vi "get_speeds_and_positions.vi"(1 "error in (no error)":errorcluster) -> (0 "error out":errorcluster)   [LabVIEW 2016]
uses:
  sa commands.ctl
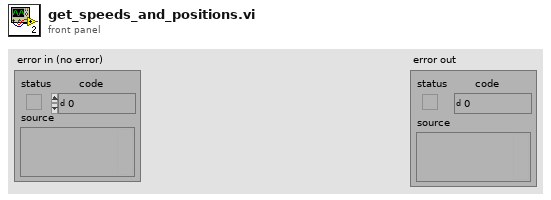
[diagram p1: front panel]
types:
  T1 = typedef "sa commands.ctl" = enum16{"read all", "set system index", "set x channel", "set y channel", "set rotation channel"}
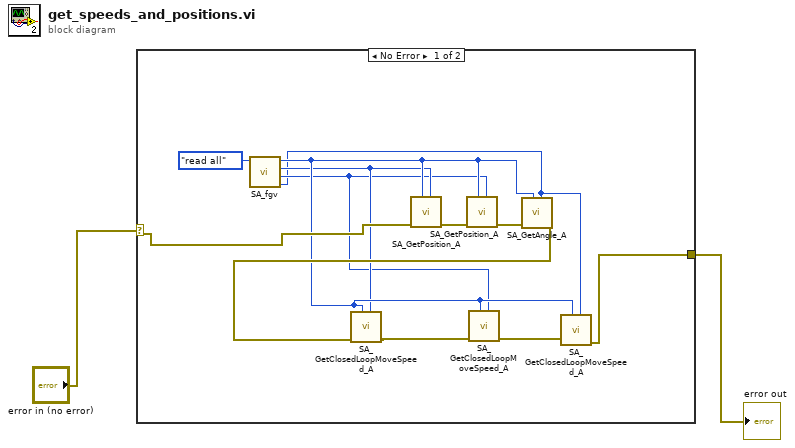
[diagram p0: block diagram]
diagram:
  n1 = case shown="No Error" "error in (no error)" {
    selector: "error in (no error)" -> [w11 w15]
    tunnel: [w3 w15] -> w1
    frame No Error {
      n2 = call "SA_fgv.vi"("command"=sa_commands."read all") -> ("rotation channel"=w4:u32, "y channel"=w5:u32, "x channel"=w6:u32, "system index"=w7:u32)  [unwired: 3 in]
      n3 = call <vilib>:"SA_GetPosition_A.vi"("channelIndex"=w6, "systemIndex"=w7, "error in (no error)"=w11) -> ("error out"=w10:errorcluster)  [unwired: 8 in]
      n4 = call <vilib>:"SA_GetPosition_A.vi"("channelIndex"=w5, "systemIndex"=w7, "error in (no error)"=w10) -> ("error out"=w9:errorcluster)  [unwired: 8 in]
      n5 = call <vilib>:"SA_GetAngle_A.vi"("channelIndex"=w4, "systemIndex"=w7, "error in (no error)"=w9) -> ("error out"=w8:errorcluster)  [unwired: 8 in]
      n6 = call <vilib>:"SA_GetClosedLoopMoveSpeed_A.vi"("channelIndex"=w6, "systemIndex"=w7, "error in (no error)"=w8) -> ("error out"=w12:errorcluster)  [unwired: 8 in]
      n7 = call <vilib>:"SA_GetClosedLoopMoveSpeed_A.vi"("channelIndex"=w5, "systemIndex"=w7, "error in (no error)"=w12) -> ("error out"=w13:errorcluster)  [unwired: 8 in]
      n8 = call <vilib>:"SA_GetClosedLoopMoveSpeed_A.vi"("channelIndex"=w4, "systemIndex"=w7, "error in (no error)"=w13) -> ("error out"=w3:errorcluster)  [unwired: 8 in]
    }
    frame Error {
    }
  }
  "error out" <- w1
